vi "TLB Native Dynamic Events ver 0.05c.vi"() -> ()   [LabVIEW 2018]
uses:
  Labview Training Phase 2/Enum Controls/States for Action Engine.ctl
  Type def/TLB event states.ctl
  Type def/TLB MHL States.ctl
  <vilib>/Studica/Studica Toolkit/Background/I2C Channel.ctl
  <vilib>/Studica/Studica Toolkit/NavX/NavX.lvlib
  <vilib>/myRIO/Common/Instrument Driver Framework/myRIO v1.0/AI/typedefs/AI Channels Enum.ctl
  <vilib>/myRIO/Common/Instrument Driver Framework/myRIO v1.0/AI/typedefs/AI Channels List.ctl
  <vilib>/Studica/Studica Toolkit/Background/Mxp Selection.ctl
  <vilib>/ptbypt/NI_PtbyPt.lvlib
  Type def/Type def.ctl
panel:
  out "Object detected":bool
  out "Yaw":dbl
  in  "NavX Zero Yaw":bool
  out "NavX Info Out":T2
  out "LinearAcceleration":T3
  out "Displacement":T4
  out "YRPHfH":T5
  in  "y":dbl=-1.2 format="%#_13g"
  out "Distance":T6
  in  "Return to IDLE":bool
  out "Right IR Sensor":dbl
  out "Left IR Sensor":dbl
  out "CM":fxp<+,64,16>
  out "Ultrasonic sensor":dbl format="%0.2f"
  in  "xTargetSpeed":dbl
  in  "yTargetSpeed":dbl
  in  "wTargetSpeed":dbl
  out "Speed":T7
  in  "Reset Encoder 0":bool
  out "Action Queue Items":i32
  out "State Logic Queue Items":i32
  out "Action Queues items":string[](array[string])=["Hardware reset", "Software reset", ""]
  out "State logic":T8=enum."Task 2"
  out "Action State":string
  in  "Tasks Selector":string(combo)="Task 2"
  in  "Stop Queue":bool
  in  "Start Task":bool
  # "Test Programme written by Calvin Loke    Dated: 28 Aug 2019\nTest Programme revised by Dr Alex See   Dated 30 Aug 2019\n\nProgramme version:   TLB Native Dynamic Events ver 0.04b.vi"
  # "System Health Status Update"
  # "Sequence of Actions"
  # "Continuous (Repeated)"
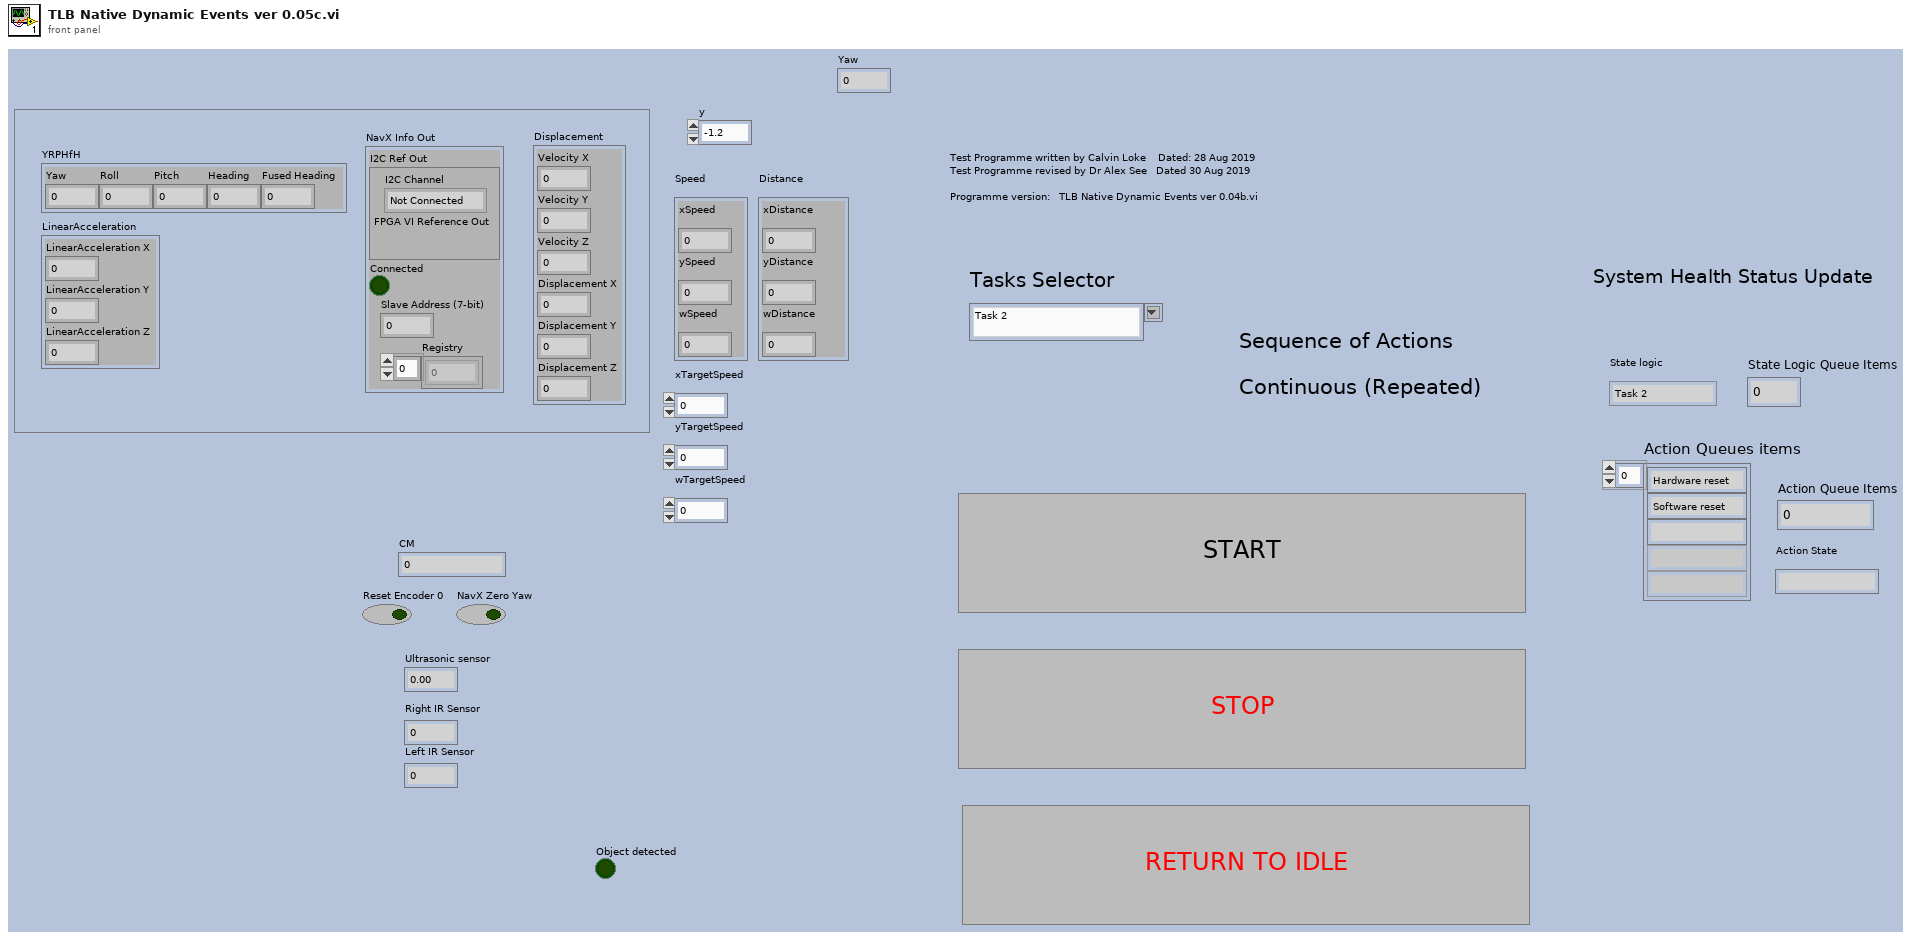
[diagram p1: front panel]
types:
  T1 = typedef "I2C Channel.ctl" = enum16{"Not Connected", "A", "B"}
  T2 = cluster{"I2C Ref Out":cluster{"I2C Channel":T1, "FPGA VI Reference Out":refnum<k20>}, "Connected":bool, "Slave Address (7-bit)":u8, "Registry":u8[]}
  T3 = cluster{"LinearAcceleration X":dbl, "LinearAcceleration Y":dbl, "LinearAcceleration Z":dbl}
  T4 = cluster{"Velocity X":dbl, "Velocity Y":dbl, "Velocity Z":dbl, "Displacement X":dbl, "Displacement Y":dbl, "Displacement Z":dbl}
  T5 = cluster{"Yaw":dbl, "Roll":dbl, "Pitch":dbl, "Heading":dbl, "Fused Heading":dbl}
  T6 = cluster{"xDistance":dbl, "yDistance":dbl, "wDistance":dbl}
  T7 = cluster{"xSpeed":dbl, "ySpeed":dbl, "wSpeed":dbl}
  T8 = typedef "TLB MHL States.ctl" = enum16{"None", "Startup", "Idle", "Processing", "Shutdown", "Reset", "Task 1", "Task 2", "Task 3", "Task 4", "Task 4a", "Task 4b", "Task 4c", "Task 4d", "Task 4e", "Task 4f", "Task 4g", "Task 4h", "Acquire image", "Wall follow mode", "Drive Straight"}
  T9 = typedef "States for Action Engine.ctl" = enum16{"Initialize", "Write", "Read"}
  T10 = typedef "Type def.ctl" = cluster{"Object detected":bool, "L IR Sensor":dbl, "In move state?":bool}
  T11 = typedef "TLB event states.ctl" = enum16{"Start Sequence", "Exit", "Start Task 1", "Start Task 2", "Start Task 3", "Start Task 4", "Camera vision", "Wall follow mode", "Idle", "Start Drive Straight"}
  T12 = typedef "Mxp Selection.ctl" = enum16{"MXP A", "MXP B"}
  T13 = typedef "AI Channels List.ctl" = T14[]
  T14 = typedef "AI Channels Enum.ctl" = enum16{"Not Connected", "AudioIn/Left", "AudioIn/Right", "C/AI0", "C/AI1", "A/AI0", "A/AI1", "A/AI2", "A/AI3", "A/AI4", "A/AI5", "A/AI6", "A/AI7", "B/AI0", "B/AI1", "B/AI2", "B/AI3", "B/AI4", "B/AI5", "B/AI6", "B/AI7", "AI/AI0", "AI/AI1", "AI/AI2", "AI/AI3", "A/AI0 (DIFF)", "A/AI1 (DIFF)", "A/AI2 (DIFF)", "A/AI3 (DIFF)", "B/AI0 (DIFF)", "B/AI1 (DIFF)", "B/AI2 (DIFF)", "B/AI3 (DIFF)"}
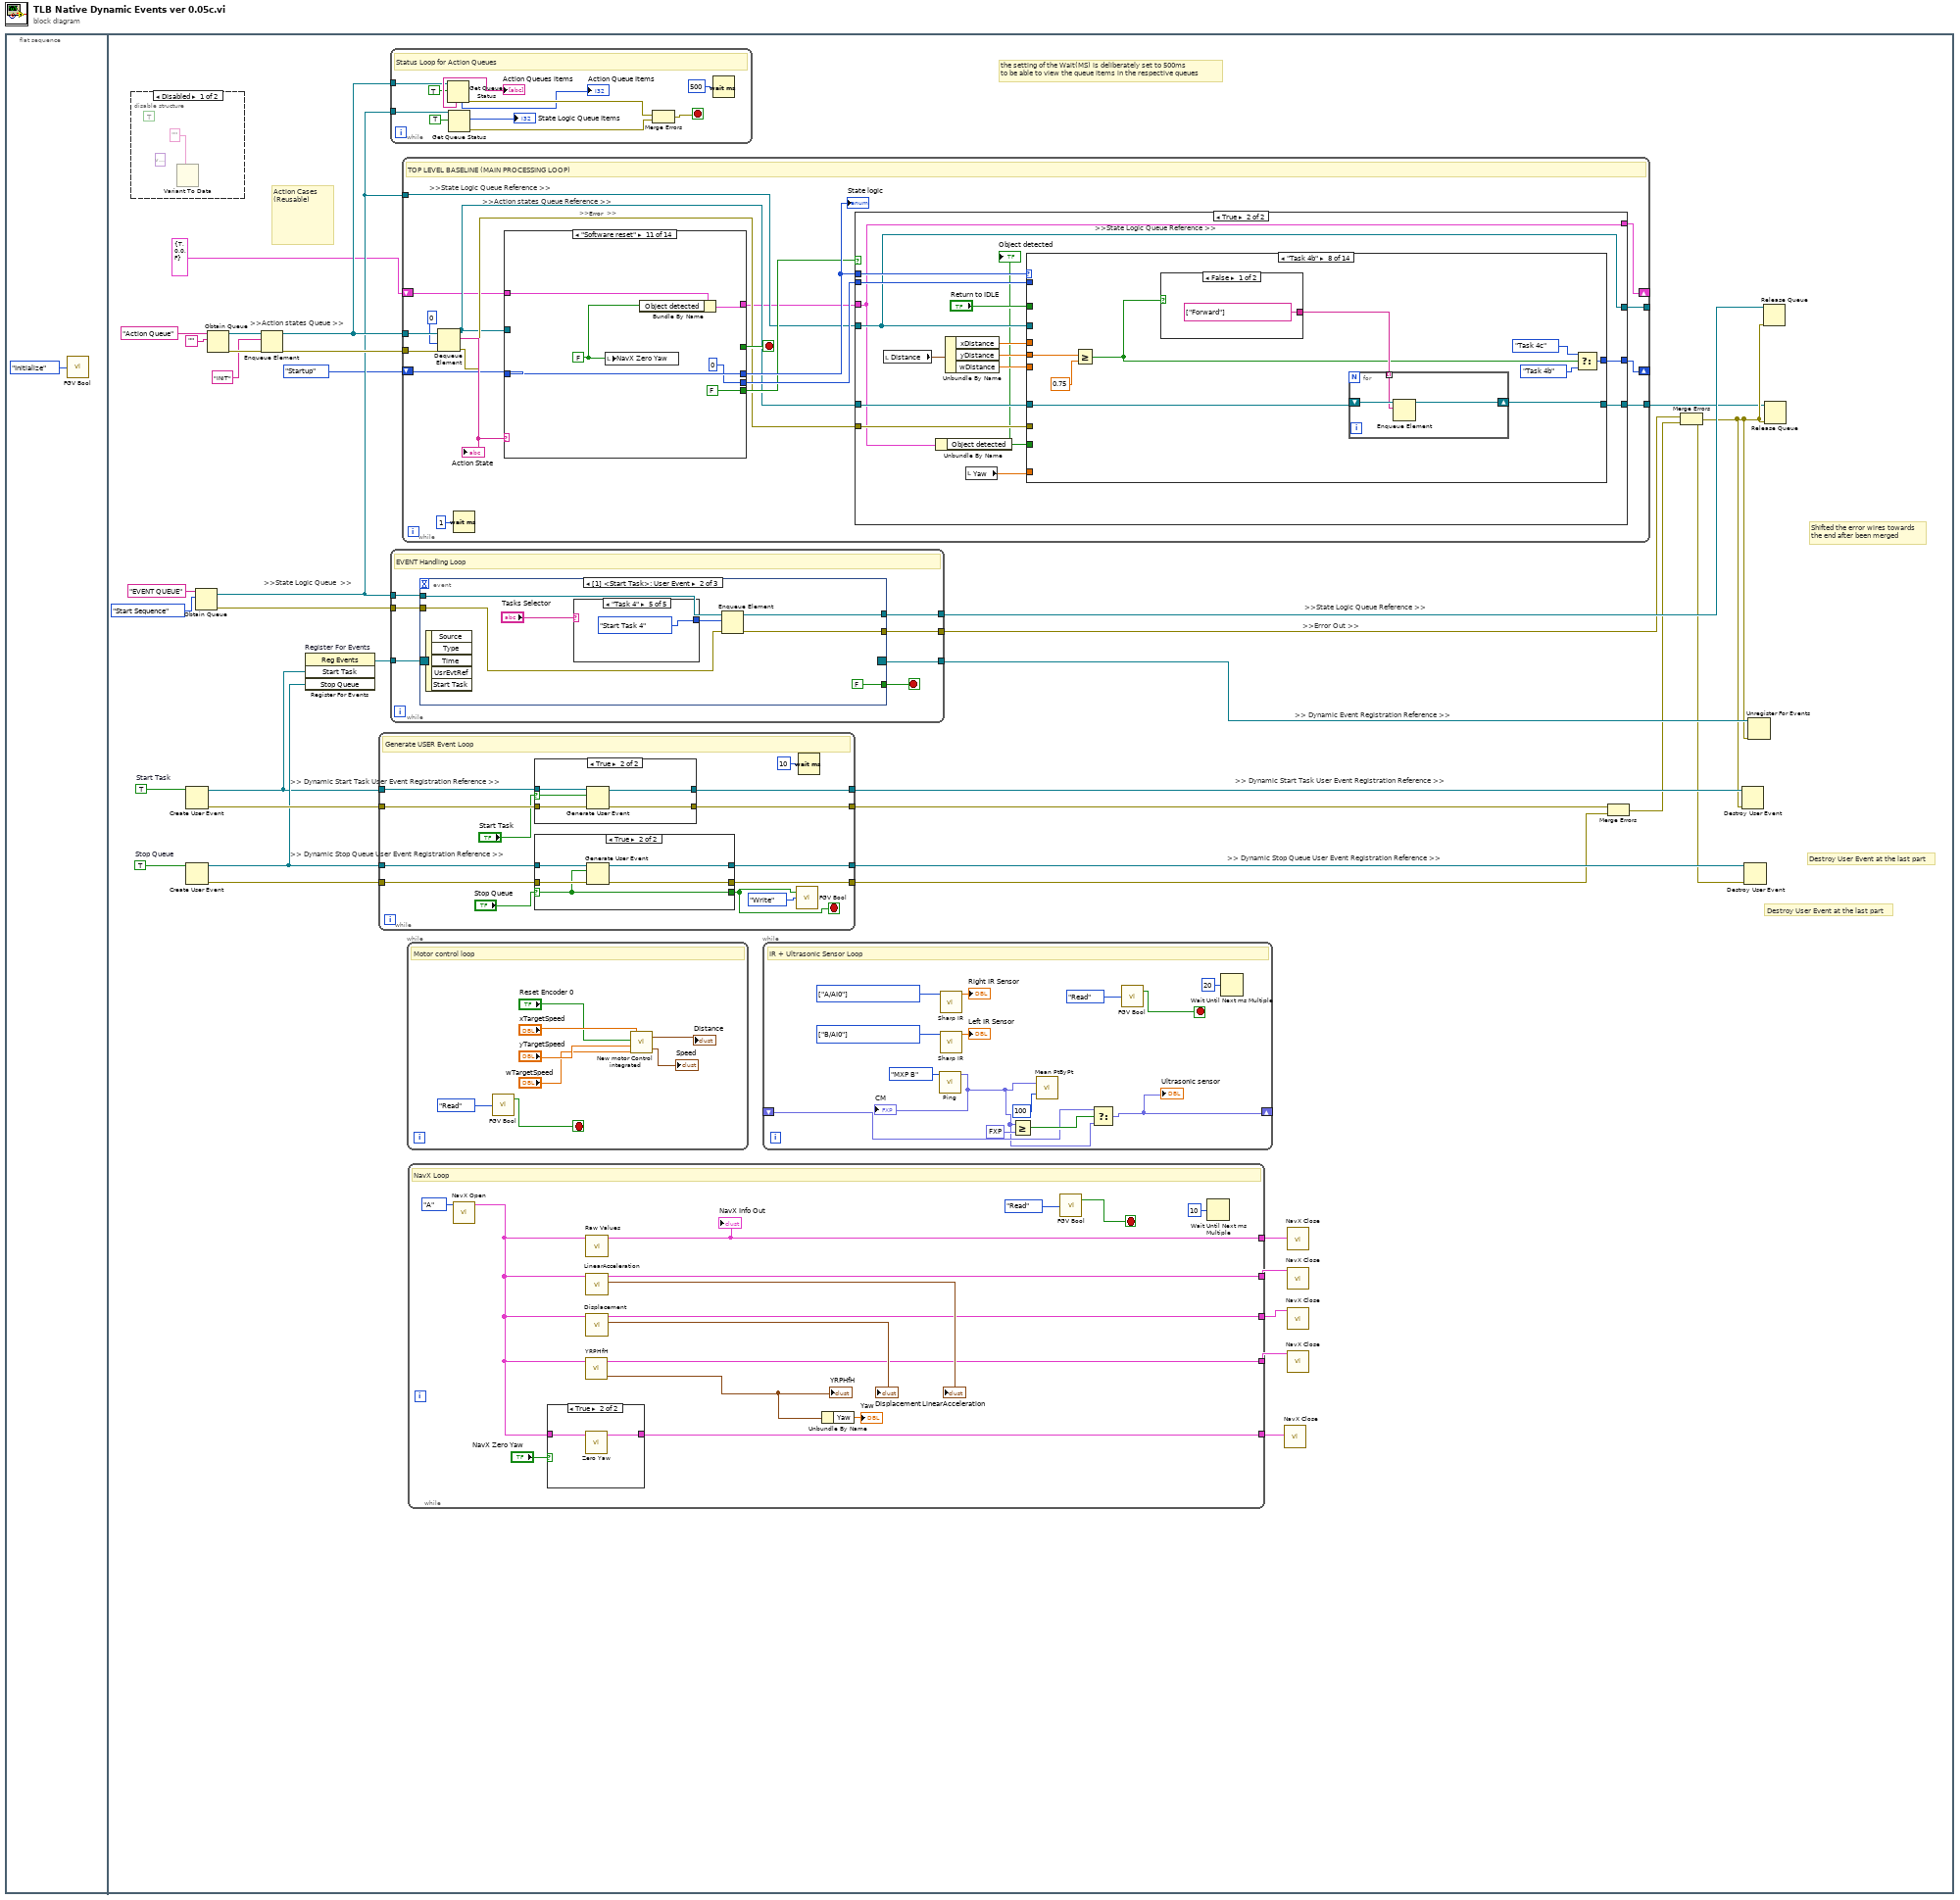
[diagram p0: block diagram]
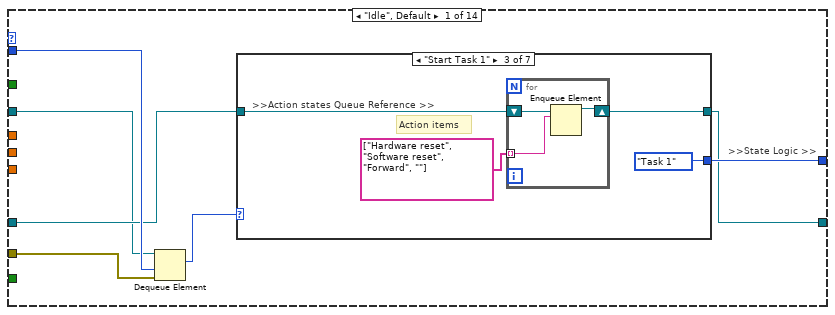
[diagram p5: hidden frame]
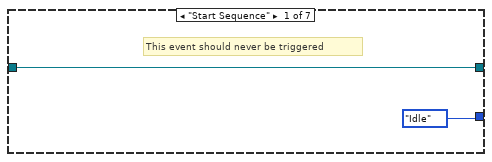
[diagram p6: hidden frame]
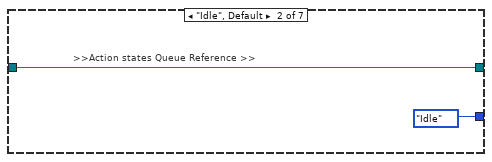
[diagram p7: hidden frame]
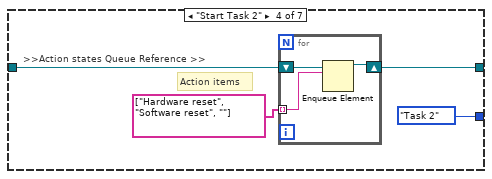
[diagram p8: hidden frame]
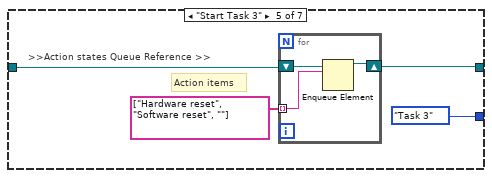
[diagram p9: hidden frame]
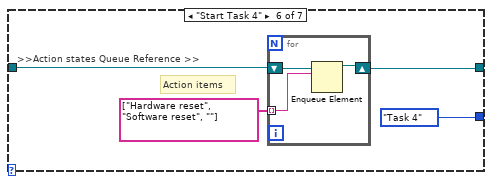
[diagram p10: hidden frame]
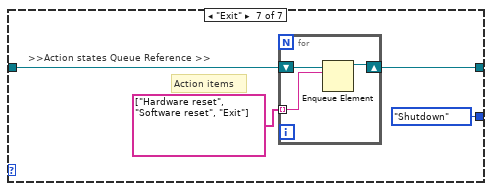
[diagram p11: hidden frame]
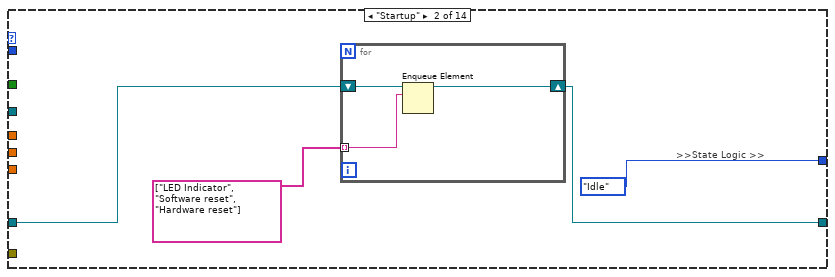
[diagram p12: hidden frame]
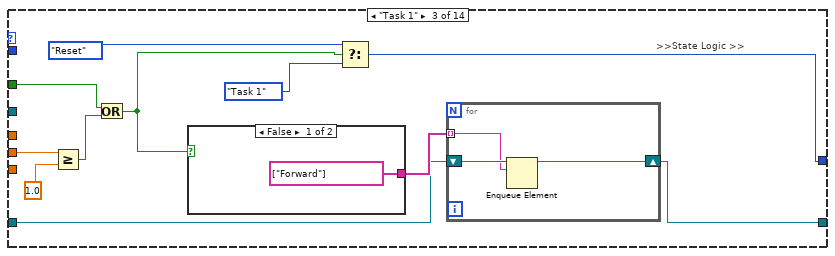
[diagram p13: hidden frame]
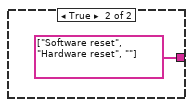
[diagram p14: hidden frame]
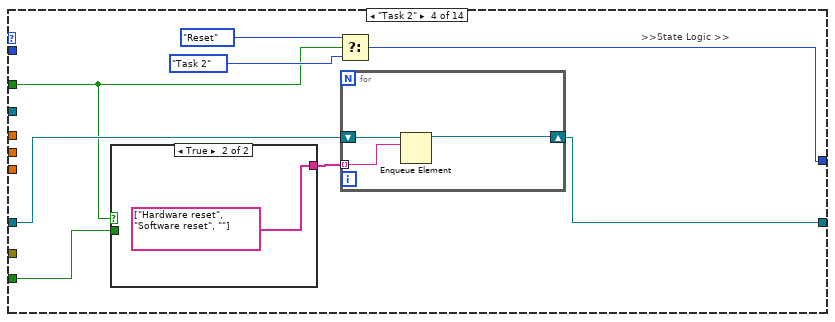
[diagram p15: hidden frame]
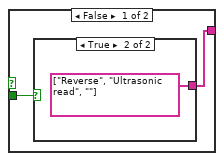
[diagram p16: hidden frame]
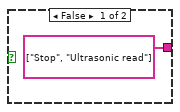
[diagram p17: hidden frame]
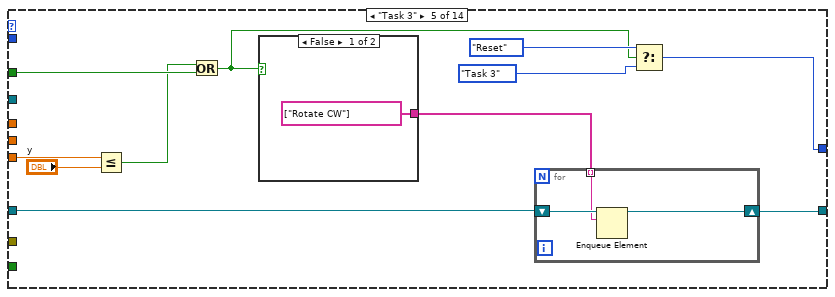
[diagram p18: hidden frame]
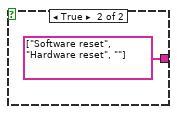
[diagram p19: hidden frame]
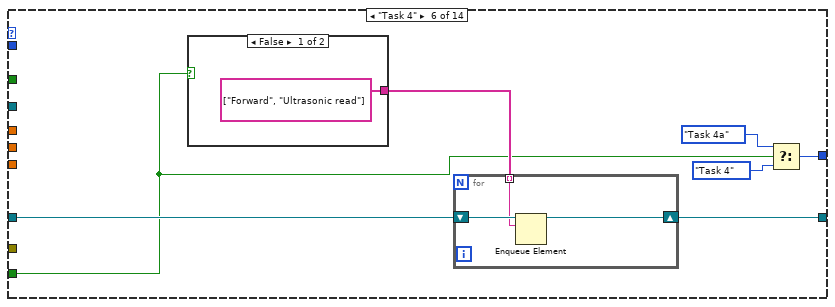
[diagram p20: hidden frame]
diagram:
  n1 = flat-sequence {
    frame #0 {
      n2 = call "FGV Bool.vi"("Init/Read/Write State"=States_for_Action_Engine."Initialize") -> ()  [unwired: 2 in, 2 out]
    }
    frame #1 {
      w36 = TRUE  # Stop Queue
      w35 = TRUE  # Start Task
      # "the setting of the Wait(MS) is deliberately set to 500ms\nto be able to view the queue items in the respective queues"
      # "Action Cases\n(Reusable)"
      # ">>Error Out >>"
      # ">> Dynamic Stop Queue User Event Registration Reference >>"
      # ">> Dynamic Start Task User Event Registration Reference >>"
      # ">> Dynamic Stop Queue User Event Registration Reference >>"
      # ">> Dynamic Start Task User Event Registration Reference >>"
      # ">> Dynamic Event Registration Reference >>"
      # ">>Action states Queue >>"
      # ">>State Logic Queue  >>"
      # ">>State Logic Queue Reference >>"
      # "Destroy User Event at the last part"
      # "Destroy User Event at the last part"
      # "Shifted the error wires towards\nthe end after been merged"
      n3 = disable-structure shown="Disabled" {
        frame Disabled {
          (unwired) variant
          (unwired) TRUE
          n4 = Variant To Data(type="") -> ()  [unwired: 2 in, 2 out]
        }
        frame Enabled {
        }
      }
      n5 = Create User Event(user event datatype=w35) -> (user event=w27:refnum<user-event>, error out=w32:errorcluster)  [unwired: 1 in]
      n6 = Create User Event(user event datatype=w36) -> (user event=w28:refnum<user-event>, error out=w31:errorcluster)  [unwired: 1 in]
      n7 = Obtain Queue(name (unnamed)="EVENT QUEUE", element data type=TLB_event_states."Start Sequence" ("Enum")) -> (queue out=w12:refnum<queue>, error out=w18:errorcluster)  [unwired: 3 in, 1 out]
      n8 = Obtain Queue(name (unnamed)="Action Queue", element data type="") -> (queue out=w21:refnum<queue>, error out=w17:errorcluster)  [unwired: 3 in, 1 out]
      n9 = Enqueue Element(queue=w21, element="INIT", error in (no error)=w17) -> (queue out=w13:refnum<queue>, error out=w16:errorcluster)  [unwired: 1 in, 1 out]
      n10 = register-events "Register For Events"(w27, w28) -> (reference out=w26:refnum<event-registration>)  [unwired: 2 in, 1 out]
      n11 = while {
        tunnel: w27 -> [w453]
        tunnel: w28 -> [w452]
        tunnel: [w451] -> w34
        tunnel: [w450] -> w33
        tunnel: w32 -> [w449]
        tunnel: [w448] -> w30
        tunnel: w31 -> [w447]
        tunnel: [w446] -> w29
        stop <- w442 stop-if-true
        # "Generate USER Event Loop"
        n12 = case shown="True" "Start Task" {
          selector: "Start Task" -> [_ w465]
          tunnel: w453 -> [w464 w469]
          tunnel: [w464 w468] -> w450
          tunnel: w449 -> [w463 w467]
          tunnel: [w463 w466] -> w448
          frame False {
          }
          frame True {
            n13 = Generate User Event(user event=w469, event data cluster=w465, error in=w467) -> (user event out=w468:refnum<user-event>, error out=w466:errorcluster)  [unwired: 1 in]
          }
        }
        n14 = case shown="True" "Stop Queue" {
          selector: "Stop Queue" -> [_ w458]
          tunnel: w452 -> [w457 w462]
          tunnel: [w457 w461] -> w451
          tunnel: w447 -> [w456 w460]
          tunnel: [w456 w459] -> w446
          tunnel: [FALSE w458] -> w442
          frame False {
          }
          frame True {
            n15 = Generate User Event(user event=w462, event data cluster=w458, error in=w460) -> (user event out=w461:refnum<user-event>, error out=w459:errorcluster)  [unwired: 1 in]
          }
        }
        n16 = call "FGV Bool.vi"("Init/Read/Write State"=States_for_Action_Engine."Write", "Input Node"=w442) -> ()  [unwired: 1 in, 2 out]
        n17 = Wait (ms)(milliseconds to wait=u32 10) -> ()  [unwired: 1 out]
      }
      n18 = while {
        tunnel: w13 -> [w86]
        tunnel: w12 -> [w83]
        stop <- w80 stop-if-true
        # "Status Loop for Action Queues"
        n19 = Get Queue Status(queue=w86, return elements? (F)=TRUE) -> (error out=w82:errorcluster, # elements in queue=→"Action Queue Items":i32, elements=→"Action Queues items":string[])  [unwired: 1 in, 5 out]
        n20 = Get Queue Status(queue=w83, return elements? (F)=TRUE) -> (# pending remove=→"State Logic Queue Items":i32, error out=w81:errorcluster)  [unwired: 1 in, 6 out]
        n21 = Merge Errors(w82, w81) -> (w80:errorcluster)
        n22 = Wait (ms)(milliseconds to wait=u32 500) -> ()  [unwired: 1 out]
      }
      n23 = while {
        tunnel: w26 -> [w417]
        tunnel: [w416] -> w25
        tunnel: w12 -> [w414]
        tunnel: [w413] -> w24
        tunnel: w18 -> [w412]
        tunnel: [w411] -> w15
        stop <- w415 stop-if-true
        # "EVENT Handling Loop"
        n24 = event shown="[1] <Start Task>: User Event" {
          selector: w417 -> [_ _ _]
          dyn-events: [_ _ _] -> w416
          timeout: _ -> [_ _ _]
          tunnel: [FALSE FALSE w441] -> w415
          tunnel: w414 -> [w422 w429 w439]
          tunnel: [w421 w428 w440] -> w413
          tunnel: w412 -> [w419 w425 w437]
          tunnel: [w418 w424 w436] -> w411
          event Timeout {
            n25 = event-data() -> ()  [unwired: 1 in, 3 out]
            n26 = Enqueue Element(queue=w422, element=TLB_event_states."Idle" ("Enum"), error in (no error)=w419) -> (queue out=w421:refnum<queue>, error out=w418:errorcluster)  [unwired: 1 in, 1 out]
          }
          event User Event {
            n27 = event-data() -> ()  [unwired: 1 in, 5 out]
            n28 = case shown="\"Task 4\"" "Tasks Selector" {
              tunnel: [TLB_event_states."Idle" ("Enum") TLB_event_states."Start Task 1" ("Enum") TLB_event_states."Start Task 2" ("Enum") TLB_event_states."Start Task 3" ("Enum") TLB_event_states."Start Task 4" ("Enum")] -> w426
              frame Default {
              }
              frame "Task 1" {
              }
              frame "Task 2" {
              }
              frame "Task 3" {
              }
              frame "Task 4" {
              }
            }
            n29 = Enqueue Element(queue=w429, element=w426, error in (no error)=w425) -> (queue out=w428:refnum<queue>, error out=w424:errorcluster)  [unwired: 1 in, 1 out]
          }
          event User Event {
            n30 = event-data() -> ("Stop Queue"=w441:bool)  [unwired: 1 in, 4 out]
            n31 = Enqueue Element At Opposite End(queue=w439, element=TLB_event_states."Exit" ("Enum"), error in (no error)=w437) -> (queue out=w440:refnum<queue>, error out=w436:errorcluster)  [unwired: 1 in, 1 out]
          }
        }
      }
      n32 = while {
        tunnel: w12 -> [w95]
        shift-right: [w100] -> _
        shift-left: TLB_MHL_States."Startup" ("Enum") -> [w92]
        tunnel: w13 -> [w105]
        tunnel: w16 -> [w103]
        tunnel: [w102] -> _
        tunnel: [w101] -> w10
        shift-right: [w89] -> _
        shift-left: T10 {"Object detected"=TRUE, "L IR Sensor"=0.0, "In move state?"=FALSE} -> [w91]
        stop <- w98 stop-if-true
        # ">>Error  >>"
        # ">>Action states Queue Reference >>"
        # ">>State Logic Queue Reference >>"
        # "TOP LEVEL BASELINE (MAIN PROCESSING LOOP)"
        n33 = Dequeue Element(queue=w105, timeout in ms (-1)=0, error in (no error)=w103) -> (queue out=w93:refnum<queue>, element=w104:string, error out=w94:errorcluster)  [unwired: 1 out]
        "Action State" <- w104
        n34 = Wait (ms)(milliseconds to wait=u32 1) -> ()  [unwired: 1 out]
        n35 = case shown="\"Software reset\"" w104 {
          tunnel: [w314 w320 w324 w331 w340 w348 w354 w364 w371 w378 w385 w392 TLB_MHL_States."Shutdown" ("Enum") w410] -> w106
          tunnel: [w313 0 0 0 0 0 0 0 0 0 0 0 0 0] -> w99
          tunnel: [_ _ _ _ _ _ _ _ _ _ _ _ TRUE _] -> w98
          tunnel: [TRUE FALSE FALSE FALSE FALSE FALSE FALSE FALSE FALSE FALSE FALSE FALSE FALSE FALSE] -> w97
          tunnel: w93 -> [_ _ _ _ _ _ _ _ _ _ _ _ _ _]
          tunnel: w92 -> [w314 w320 w324 w331 w340 w348 w354 w364 w371 w378 w385 w392 _ w410]
          tunnel: w91 -> [w311 w317 w321 w325 w333 w341 w349 w357 w365 w373 w382 w386 w393 w409]
          tunnel: [w311 w317 w321 w325 w333 w341 w349 w357 w365 w373 w381 w386 w393 w404] -> w90
          frame "No action", Default {
            n36 = case shown="\"Idle\"" w314 {
              tunnel: [0 100] -> w313
              frame "Startup", Default {
              }
              frame "Idle" {
              }
            }
          }
          frame "Init" {
            # ">>State Logic  >>"
          }
          frame "LED Indicator" {
          }
          frame "Forward" {
            w327 = 0.0
            n37 = local write "NavX Zero Yaw"(FALSE ("NavX Zero Yaw")) -> ()
            n38 = local write "Reset Encoder 0"(FALSE ("Reset Encoder 0")) -> ()
            n39 = local write "wTargetSpeed"(w327) -> ()
            n40 = local write "yTargetSpeed"(0.5 ("yTargetSpeed")) -> ()
            n41 = local write "xTargetSpeed"(w327) -> ()
          }
          frame "Right" {
            w335 = 0.0
            n42 = local write "NavX Zero Yaw"(FALSE ("NavX Zero Yaw")) -> ()
            n43 = local write "Reset Encoder 0"(FALSE ("Reset Encoder 0")) -> ()
            n44 = local write "wTargetSpeed"(w335) -> ()
            n45 = local write "yTargetSpeed"(w335) -> ()
            n46 = local write "xTargetSpeed"(0.5 ("yTargetSpeed")) -> ()
          }
          frame "Left" {
            w343 = 0.0
            n47 = local write "NavX Zero Yaw"(FALSE ("NavX Zero Yaw")) -> ()
            n48 = local write "Reset Encoder 0"(FALSE ("Reset Encoder 0")) -> ()
            n49 = local write "wTargetSpeed"(w343) -> ()
            n50 = local write "yTargetSpeed"(w343) -> ()
            n51 = local write "xTargetSpeed"(-0.5 ("yTargetSpeed")) -> ()
          }
          frame "Rotate CW" {
            w351 = 0.0
            n52 = local write "NavX Zero Yaw"(FALSE ("NavX Zero Yaw")) -> ()
            n53 = local write "Reset Encoder 0"(FALSE ("Reset Encoder 0")) -> ()
            n54 = local write "wTargetSpeed"(-0.15 ("yTargetSpeed")) -> ()
            n55 = local write "yTargetSpeed"(w351) -> ()
            n56 = local write "xTargetSpeed"(w351) -> ()
          }
          frame "Rotate ACW" {
            w361 = 0.0
            n57 = local write "NavX Zero Yaw"(FALSE ("NavX Zero Yaw")) -> ()
            n58 = local write "Reset Encoder 0"(FALSE ("Reset Encoder 0")) -> ()
            n59 = local write "wTargetSpeed"(0.15 ("yTargetSpeed")) -> ()
            n60 = local write "yTargetSpeed"(w361) -> ()
            n61 = local write "xTargetSpeed"(w361) -> ()
          }
          frame "Reverse" {
            w367 = 0.0
            n62 = local write "NavX Zero Yaw"(FALSE ("NavX Zero Yaw")) -> ()
            n63 = local write "wTargetSpeed"(w367) -> ()
            n64 = local write "yTargetSpeed"(-0.3 ("yTargetSpeed")) -> ()
            n65 = local write "xTargetSpeed"(w367) -> ()
            n66 = local write "Reset Encoder 0"(FALSE ("Reset Encoder 0")) -> ()
          }
          frame "Stop" {
            w375 = 0.0
            n67 = local write "NavX Zero Yaw"(FALSE ("NavX Zero Yaw")) -> ()
            n68 = local write "wTargetSpeed"(w375) -> ()
            n69 = local write "yTargetSpeed"(w375) -> ()
            n70 = local write "xTargetSpeed"(w375) -> ()
            n71 = local write "Reset Encoder 0"(FALSE ("Reset Encoder 0")) -> ()
          }
          frame "Software reset" {
            w380 = FALSE ("NavX Zero Yaw")
            n72 = local write "NavX Zero Yaw"(w380) -> ()
            n73 = Bundle By Name(cluster=w382, "Object detected"=w380) -> (w381:T10)
          }
          frame "Hardware reset" {
            w388 = 0.0
            n74 = local write "NavX Zero Yaw"(TRUE ("NavX Zero Yaw")) -> ()
            n75 = local write "Reset Encoder 0"(TRUE ("Reset Encoder 0")) -> ()
            n76 = local write "wTargetSpeed"(w388) -> ()
            n77 = local write "yTargetSpeed"(w388) -> ()
            n78 = local write "xTargetSpeed"(w388) -> ()
          }
          frame "Exit" {
          }
          frame "Ultrasonic read" {
            n79 = local read "Left IR Sensor"() -> (w403:dbl)
            n80 = local read "Ultrasonic sensor"() -> (w401:dbl)
            n81 = Greater?(x=w401, y=10.0) -> (0:w399:bool)
            n82 = Greater?(x=w403, y=20.0) -> (0:w398:bool)
            n83 = Less?(x=w401, y=40.0) -> (x < y?=w405:bool)
            n84 = And(x=w399, y=w398) -> ()  [unwired: 1 out]
            n85 = Bundle By Name(cluster=w409, "Object detected"=w405) -> (w404:T10)
          }
        }
        "State logic" <- w106
        n86 = case shown="True" w97 {
          tunnel: w106 -> [w110 w126]
          tunnel: w95 -> [w111 w120]
          tunnel: w93 -> [w109 w125]
          tunnel: [w111 w120] -> w102
          tunnel: [w109 w124] -> w101
          tunnel: [w110 w123] -> w100
          tunnel: w94 -> [_ w122]
          tunnel: w99 -> [_ w121]
          tunnel: w90 -> [w108 w112]
          tunnel: [w108 w112] -> w89
          frame False {
          }
          frame True {
            # ">>State Logic Queue Reference >>"
            n87 = local read "Distance"() -> (w118:T6)
            n88 = Unbundle By Name(w112) -> ("Object detected"=w113:bool)
            "Object detected" <- w113
            n89 = Unbundle By Name(w118) -> ("xDistance"=w115:dbl, "yDistance"=w117:dbl, "wDistance"=w116:dbl)
            n90 = local read "Yaw"() -> (w114:dbl)
            n91 = case shown="\"Task 4b\"" w126 {
              tunnel: w120 -> [w127 _ _ _ _ _ _ _ _ _ _ _ _ _]
              tunnel: w125 -> [w129 w174 w186 w199 w221 w230 w242 w257 w270 w283 w294 w300 w303 w309]
              tunnel: [w128 w173 w185 w200 w220 w231 w241 w256 w269 w282 w293 w300 w302 w309] -> w124
              tunnel: [w132 TLB_MHL_States."Idle" ("Enum") w188 w201 w217 w234 w244 w255 w271 w281 TLB_MHL_States."Idle" ("Enum") TLB_MHL_States."Reset" ("Enum") TLB_MHL_States."Shutdown" ("Enum") TLB_MHL_States."Reset" ("Enum")] -> w123
              tunnel: w122 -> [w130 _ _ _ _ _ _ _ _ _ _ _ _ _]
              tunnel: w121 -> [w131 _ _ _ _ _ _ _ _ _ _ _ _ _]
              tunnel: "Return to IDLE" -> [_ _ w183 w198 w215 _ _ _ _ _ _ _ _ _]
              tunnel: w117 -> [_ _ w182 _ _ _ _ w254 _ _ _ _ _ _]
              tunnel: w116 -> [_ _ _ _ w214 _ _ _ _ _ _ _ _ _]
              tunnel: w115 -> [_ _ _ _ _ _ _ _ w266 _ _ _ _ _]
              tunnel: w114 -> [_ _ _ _ _ _ _ _ _ _ _ _ _ _]
              tunnel: w113 -> [_ _ _ w196 _ w228 w240 _ _ w280 _ _ _ _]
              frame "Idle", Default {
                # ">>State Logic >>"
                n92 = Dequeue Element(queue=w127, timeout in ms (-1)=w131, error in (no error)=w130) -> (element=w133:T11)  [unwired: 3 out]
                n93 = case shown="\"Start Task 1\"" w133 {
                  tunnel: [TLB_MHL_States."Idle" ("Enum") TLB_MHL_States."Idle" ("Enum") TLB_MHL_States."Task 1" ("Enum") TLB_MHL_States."Task 2" ("Enum") TLB_MHL_States."Task 3" ("Enum") TLB_MHL_States."Task 4" ("Enum") TLB_MHL_States."Shutdown" ("Enum")] -> w132
                  tunnel: [w135 w136 w140 w145 w154 w160 w166] -> w128
                  tunnel: w129 -> [w135 w136 w138 w146 w155 w161 w167]
                  frame "Start Sequence" {
                    # "This event should never be triggered"
                  }
                  frame "Idle", Default {
                    # ">>Action states Queue Reference >>"
                  }
                  frame "Start Task 1" {
                    # ">>Action states Queue Reference >>"
                    # "Action items"
                    n94 = for {
                      shift-right: [w144] -> w140
                      shift-left: w138 -> [w143]
                      tunnel: string[] ["Hardware reset", "Software reset", "Forward", ""] -> [w142] mode=indexing
                      n95 = Enqueue Element(queue=w143, element=w142) -> (queue out=w144:refnum<queue>)  [unwired: 2 in, 2 out]
                    }
                  }
                  frame "Start Task 2" {
                    # ">>Action states Queue Reference >>"
                    # "Action items"
                    n96 = for {
                      shift-right: [w151] -> w145
                      shift-left: w146 -> [w150]
                      tunnel: string[] ["Hardware reset", "Software reset", ""] -> [w149] mode=indexing
                      n97 = Enqueue Element(queue=w150, element=w149) -> (queue out=w151:refnum<queue>)  [unwired: 2 in, 2 out]
                    }
                  }
                  frame "Start Task 3" {
                    # ">>Action states Queue Reference >>"
                    # "Action items"
                    n98 = for {
                      shift-right: [w158] -> w154
                      shift-left: w155 -> [w157]
                      tunnel: string[] ["Hardware reset", "Software reset", ""] -> [w156] mode=indexing
                      n99 = Enqueue Element(queue=w157, element=w156) -> (queue out=w158:refnum<queue>)  [unwired: 2 in, 2 out]
                    }
                  }
                  frame "Start Task 4" {
                    # ">>Action states Queue Reference >>"
                    # "Action items"
                    n100 = for {
                      shift-right: [w165] -> w160
                      shift-left: w161 -> [w164]
                      tunnel: string[] ["Hardware reset", "Software reset", ""] -> [w163] mode=indexing
                      n101 = Enqueue Element(queue=w164, element=w163) -> (queue out=w165:refnum<queue>)  [unwired: 2 in, 2 out]
                    }
                  }
                  frame "Exit" {
                    # ">>Action states Queue Reference >>"
                    # "Action items"
                    n102 = for {
                      shift-right: [w172] -> w166
                      shift-left: w167 -> [w171]
                      tunnel: string[] ["Hardware reset", "Software reset", "Exit"] -> [w170] mode=indexing
                      n103 = Enqueue Element(queue=w171, element=w170) -> (queue out=w172:refnum<queue>)  [unwired: 2 in, 2 out]
                    }
                  }
                }
              }
              frame "Startup" {
                # ">>State Logic >>"
                n104 = for {
                  shift-right: [w178] -> w173
                  shift-left: w174 -> [w179]
                  tunnel: string[] ["LED Indicator", "Software reset", "Hardware reset"] -> [w177] mode=indexing
                  n105 = Enqueue Element(queue=w179, element=w177) -> (queue out=w178:refnum<queue>)  [unwired: 2 in, 2 out]
                }
              }
              frame "Task 1" {
                # ">>State Logic >>"
                n106 = Greater Or Equal?(x=w182, y=1.0) -> (x >= y?=w180:bool)
                n107 = Or(x=w183, y=w180) -> (x .or. y?=w184:bool)
                n108 = case shown="False" w184 {
                  tunnel: [string[] ["Forward"] string[] ["Software reset", "Hardware reset", ""]] -> w187
                  frame False {
                  }
                  frame True {
                  }
                }
                n109 = Select(t=TLB_MHL_States."Reset" ("Enum"), s=w184, f=TLB_MHL_States."Task 1" ("Enum")) -> (s? t:f=w188:T8)
                n110 = for {
                  shift-right: [w194] -> w185
                  shift-left: w186 -> [w195]
                  tunnel: w187 -> [w193] mode=indexing
                  n111 = Enqueue Element(queue=w195, element=w193) -> (queue out=w194:refnum<queue>)  [unwired: 2 in, 2 out]
                }
              }
              frame "Task 2" {
                # ">>State Logic >>"
                n112 = case shown="True" w198 {
                  tunnel: [w205 string[] ["Hardware reset", "Software reset", ""]] -> w197
                  tunnel: w196 -> [w204 _]
                  frame False {
                    n113 = case shown="True" w204 {
                      tunnel: [string[] ["Stop", "Ultrasonic read"] string[] ["Reverse", "Ultrasonic read", ""]] -> w205
                      frame False {
                      }
                      frame True {
                      }
                    }
                  }
                  frame True {
                  }
                }
                n114 = Select(t=TLB_MHL_States."Reset" ("Enum"), s=w198, f=TLB_MHL_States."Task 2" ("Enum")) -> (s? t:f=w201:T8)
                n115 = for {
                  shift-right: [w210] -> w200
                  shift-left: w199 -> [w211]
                  tunnel: w197 -> [w209] mode=indexing
                  n116 = Enqueue Element(queue=w211, element=w209) -> (queue out=w210:refnum<queue>)  [unwired: 2 in, 2 out]
                }
              }
              frame "Task 3" {
                n117 = Less Or Equal?(x=w214, y="y") -> (x <= y?=w212:bool)
                n118 = Or(x=w212, y=w215) -> (x .or. y?=w216:bool)
                n119 = case shown="False" w216 {
                  tunnel: [string[] ["Rotate CW"] string[] ["Software reset", "Hardware reset", ""]] -> w222
                  frame False {
                  }
                  frame True {
                  }
                }
                n120 = for {
                  shift-right: [w224] -> w220
                  shift-left: w221 -> [w225]
                  tunnel: w222 -> [w223] mode=indexing
                  n121 = Enqueue Element(queue=w225, element=w223) -> (queue out=w224:refnum<queue>)  [unwired: 2 in, 2 out]
                }
                n122 = Select(t=TLB_MHL_States."Reset" ("Enum"), s=w216, f=TLB_MHL_States."Task 3" ("Enum")) -> (s? t:f=w217:T8)
              }
              frame "Task 4" {
                n123 = case shown="False" w228 {
                  tunnel: [string[] ["Forward", "Ultrasonic read"] string[] ["Stop", "Hardware reset", "Software reset"]] -> w229
                  frame False {
                  }
                  frame True {
                  }
                }
                n124 = for {
                  shift-right: [w238] -> w231
                  shift-left: w230 -> [w239]
                  tunnel: w229 -> [w237] mode=indexing
                  n125 = Enqueue Element(queue=w239, element=w237) -> (queue out=w238:refnum<queue>)  [unwired: 2 in, 2 out]
                }
                n126 = Select(t=TLB_MHL_States."Task 4a" ("Enum"), s=w228, f=TLB_MHL_States."Task 4" ("Enum")) -> (s? t:f=w234:T8)
              }
              frame "Task 4a" {
                n127 = case shown="False" w240 {
                  tunnel: [string[] ["Right", "Ultrasonic read"] string[] ["Stop", "Hardware reset", "Software reset"]] -> w243
                  frame False {
                  }
                  frame True {
                  }
                }
                n128 = for {
                  shift-right: [w250] -> w241
                  shift-left: w242 -> [w251]
                  tunnel: w243 -> [w249] mode=indexing
                  n129 = Enqueue Element(queue=w251, element=w249) -> (queue out=w250:refnum<queue>)  [unwired: 2 in, 2 out]
                }
                n130 = Select(t=TLB_MHL_States."Task 4b" ("Enum"), s=w240, f=TLB_MHL_States."Task 4a" ("Enum")) -> (s? t:f=w244:T8)
              }
              frame "Task 4b" {
                n131 = Greater Or Equal?(x=w254, y=0.75) -> (x >= y?=w252:bool)
                n132 = case shown="False" w252 {
                  tunnel: [string[] ["Forward"] string[] ["Stop", "Hardware reset", "Software reset"]] -> w258
                  frame False {
                  }
                  frame True {
                  }
                }
                n133 = for {
                  shift-right: [w264] -> w256
                  shift-left: w257 -> [w265]
                  tunnel: w258 -> [w263] mode=indexing
                  n134 = Enqueue Element(queue=w265, element=w263) -> (queue out=w264:refnum<queue>)  [unwired: 2 in, 2 out]
                }
                n135 = Select(t=TLB_MHL_States."Task 4c" ("Enum"), s=w252, f=TLB_MHL_States."Task 4b" ("Enum")) -> (s? t:f=w255:T8)
              }
              frame "Task 4c" {
                n136 = Less Or Equal?(x=w266, y=-0.65) -> (x <= y?=w267:bool)
                n137 = case shown="False" w267 {
                  tunnel: [string[] ["Left"] string[] ["Stop", "Hardware reset", "Software reset"]] -> w272
                  frame False {
                  }
                  frame True {
                  }
                }
                n138 = for {
                  shift-right: [w278] -> w269
                  shift-left: w270 -> [w279]
                  tunnel: w272 -> [w277] mode=indexing
                  n139 = Enqueue Element(queue=w279, element=w277) -> (queue out=w278:refnum<queue>)  [unwired: 2 in, 2 out]
                }
                n140 = Select(t=TLB_MHL_States."Task 4d" ("Enum"), s=w267, f=TLB_MHL_States."Task 4c" ("Enum")) -> (s? t:f=w271:T8)
              }
              frame "Task 4d" {
                n141 = case shown="False" w280 {
                  tunnel: [string[] ["Forward", "Ultrasonic Read"] string[] ["Stop", "Hardware reset", "Software reset"]] -> w284
                  frame False {
                  }
                  frame True {
                  }
                }
                n142 = for {
                  shift-right: [w290] -> w282
                  shift-left: w283 -> [w291]
                  tunnel: w284 -> [w289] mode=indexing
                  n143 = Enqueue Element(queue=w291, element=w289) -> (queue out=w290:refnum<queue>)  [unwired: 2 in, 2 out]
                }
                n144 = Select(t=TLB_MHL_States."Task 4e" ("Enum"), s=w280, f=TLB_MHL_States."Task 4d" ("Enum")) -> (s? t:f=w281:T8)
              }
              frame "Reset" {
                n145 = for {
                  shift-right: [w298] -> w293
                  shift-left: w294 -> [w299]
                  tunnel: string[] ["Software reset", "Hardware reset", ""] -> [w297] mode=indexing
                  n146 = Enqueue Element(queue=w299, element=w297) -> (queue out=w298:refnum<queue>)  [unwired: 2 in, 2 out]
                }
                n147 = Wait (ms)(milliseconds to wait=u32 250) -> ()  [unwired: 1 out]
              }
              frame "Processing" {
              }
              frame "Shutdown" {
                # ">>State Logic >>"
                n148 = for {
                  shift-right: [w307] -> w302
                  shift-left: w303 -> [w308]
                  tunnel: string[] ["Software reset", "Hardware reset", "Exit"] -> [w306] mode=indexing
                  n149 = Enqueue Element(queue=w308, element=w306) -> (queue out=w307:refnum<queue>)  [unwired: 2 in, 2 out]
                }
              }
              frame "None" {
              }
            }
          }
        }
      }
      n150 = while {
        stop <- w76 stop-if-true
        # "Motor control loop"
        n151 = call "FGV Bool.vi"("Init/Read/Write State"=States_for_Action_Engine."Read") -> ("Output node"=w76:bool)  [unwired: 2 in, 1 out]
        n152 = call "New motor Control integrated.vi"("wTargetSpeed"="wTargetSpeed", "yTargetSpeed"="yTargetSpeed", "xTargetSpeed"="Reset Encoder 0", "Reset Encoders"="xTargetSpeed") -> ("Speed"=→"Speed":T7, "Distance"=→"Distance":T6)
      }
      n153 = while {
        tunnel: [w48] -> w6
        tunnel: [w45] -> w5
        tunnel: [w44] -> w3
        tunnel: [w43] -> w4
        tunnel: [w40] -> w2
        stop <- w50 stop-if-true
        # "NavX Loop"
        n154 = call <vilib>:"NavX Open.vi"("I2C Channel"=I2C_Channel."A") -> ("NavX Info"=w41:T2)  [unwired: 9 in, 1 out]
        n155 = case shown="True" "NavX Zero Yaw" {
          tunnel: w41 -> [w52 w54]
          tunnel: [w52 w53] -> w40
          frame False {
          }
          frame True {
            n156 = call <vilib>:"Zero Yaw.vi"("NavX Info In"=w54) -> ("NavX Info Out"=w53:T2)  [unwired: 10 in]
          }
        }
        n157 = call <vilib>:"YRPHfH.vi"("NavX Info In"=w41) -> ("YRPHfH"=w38:T5, "NavX Info Out"=w44:T2)  [unwired: 3 in]
        "YRPHfH" <- w38
        n158 = call <vilib>:"Raw Values.vi"("NavX Info In"=w41) -> ("NavX Info Out"=w48:T2)  [unwired: 8 in, 1 out]
        "NavX Info Out" <- w48
        n159 = call <vilib>:"LinearAcceleration.vi"("NavX Info In"=w41) -> ("LinearAcceleration"=→"LinearAcceleration":T3, "NavX Info Out"=w45:T2)  [unwired: 9 in]
        n160 = call <vilib>:"Displacement.vi"("NavX Info In"=w41) -> ("Displacement"=→"Displacement":T4, "NavX Info Out"=w43:T2)  [unwired: 9 in]
        n161 = Unbundle By Name(w38) -> ("Yaw"=→"Yaw":dbl)
        n162 = call "FGV Bool.vi"("Init/Read/Write State"=States_for_Action_Engine."Read") -> ("Output node"=w50:bool)  [unwired: 2 in, 1 out]
        n163 = Wait Until Next ms Multiple(millisecond multiple=u32 10) -> ()  [unwired: 1 out]
      }
      n164 = while {
        shift-right: [w56] -> _
        shift-left: _ -> [w58]
        stop <- w63 stop-if-true
        w68 = T13 [enum."B/AI0"] items=["Not Connected", "AudioIn/Left", "AudioIn/Right", "C/AI0", "C/AI1", "A/AI0", "A/AI1", "A/AI2", "A/AI3", "A/AI4", "A/AI5", "A/AI6", "A/AI7", "B/AI0", "B/AI1", "B/AI2", "B/AI3", "B/AI4", "B/AI5", "B/AI6", "B/AI7", "AI/AI0", "AI/AI1", "AI/AI2", "AI/AI3", "A/AI0 (DIFF)", "A/AI1 (DIFF)", "A/AI2 (DIFF)", "A/AI3 (DIFF)", "B/AI0 (DIFF)", "B/AI1 (DIFF)", "B/AI2 (DIFF)", "B/AI3 (DIFF)"] ("AI Channel")
        w69 = T13 [enum."A/AI0"] items=["Not Connected", "AudioIn/Left", "AudioIn/Right", "C/AI0", "C/AI1", "A/AI0", "A/AI1", "A/AI2", "A/AI3", "A/AI4", "A/AI5", "A/AI6", "A/AI7", "B/AI0", "B/AI1", "B/AI2", "B/AI3", "B/AI4", "B/AI5", "B/AI6", "B/AI7", "AI/AI0", "AI/AI1", "AI/AI2", "AI/AI3", "A/AI0 (DIFF)", "A/AI1 (DIFF)", "A/AI2 (DIFF)", "A/AI3 (DIFF)", "B/AI0 (DIFF)", "B/AI1 (DIFF)", "B/AI2 (DIFF)", "B/AI3 (DIFF)"] ("AI Channel")
        # "IR + Ultrasonic Sensor Loop"
        n165 = call <vilib>:"Ping.vi"("Mxp Side"=Mxp_Selection."MXP B") -> ("CM"=w57:fxp<+,64,16>)  [unwired: 8 in, 2 out]
        "CM" <- w57
        n166 = call <vilib>:"Sharp IR.vi"("AI Channel"=w69) -> ("Sharp IR Distance"=→"Right IR Sensor":dbl)  [unwired: 8 in, 2 out]
        n167 = call <vilib>:"Sharp IR.vi"("AI Channel"=w68) -> ("Sharp IR Distance"=→"Left IR Sensor":dbl)  [unwired: 8 in, 2 out]
        n168 = Greater Or Equal?(x=w57, y=fxp<+,64,16> 299.0) -> (x >= y?=w59:bool)
        n169 = call <vilib>:"Mean PtByPt.vi"("x"=w57, "sample length"=100) -> ()  [unwired: 2 in, 2 out]
        n170 = Select(t=w58, s=w59, f=w57) -> (s? t:f=w56:fxp<+,64,16>)
        "Ultrasonic sensor" <- w56
        n171 = call "FGV Bool.vi"("Init/Read/Write State"=States_for_Action_Engine."Read") -> ("Output node"=w63:bool)  [unwired: 2 in, 1 out]
        n172 = Wait Until Next ms Multiple(millisecond multiple=u32 20) -> ()  [unwired: 1 out]
      }
      n173 = call <vilib>:"NavX Close.vi"("NavX Info In"=w2) -> ()  [unwired: 10 in, 1 out]
      n174 = call <vilib>:"NavX Close.vi"("NavX Info In"=w6) -> ()  [unwired: 10 in, 1 out]
      n175 = call <vilib>:"NavX Close.vi"("NavX Info In"=w5) -> ()  [unwired: 10 in, 1 out]
      n176 = call <vilib>:"NavX Close.vi"("NavX Info In"=w4) -> ()  [unwired: 10 in, 1 out]
      n177 = call <vilib>:"NavX Close.vi"("NavX Info In"=w3) -> ()  [unwired: 10 in, 1 out]
      n178 = Merge Errors "Merge Errors"(w30, w29) -> (w9:errorcluster)
      n179 = Merge Errors(w15, w9) -> (w11:errorcluster)
      n180 = Destroy User Event(user event=w33, error in=w11) -> ()  [unwired: 1 out]
      n181 = Destroy User Event(user event=w34, error in=w11) -> ()  [unwired: 1 out]
      n182 = Unregister For Events(event registration refnum=w25, error in=w11) -> ()  [unwired: 1 out]
      n183 = Release Queue(queue=w24, error in (no error)=w11) -> ()  [unwired: 1 in, 3 out]
      n184 = Release Queue(queue=w10, error in (no error)=w11) -> ()  [unwired: 1 in, 3 out]
    }
  }
